vi "Configure Digital Channel.vi"(0 "ADALM2000 In":u32 caption="Instrument Handle Out", 1 "channel":u64 max=15, 2 "Trigger enable":bool, 3 "Output":bool, 4 "Digital Condition":T2, 5 "Cyclic":bool, 7 "Digital Mode":T1, 9 "Digital Delay":i64) -> (14 "ADALM2000 Out":u32 caption="Instrument Handle Out")   [LabVIEW 2015]
uses:
  Controls/DigitalTriggerCondition.ctl
  Controls/DigitalTriggerMode.ctl
  libm2k_lv.dll
panel:
  # "TRIGGER SETTINGS FOR DIO CHANNEL"
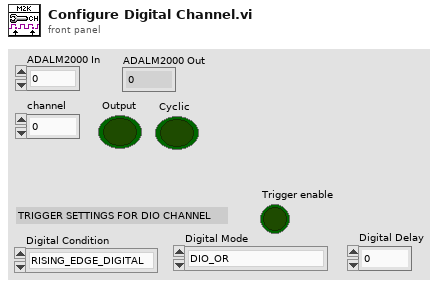
[diagram p1: front panel]
types:
  T1 = typedef "DigitalTriggerMode.ctl" = enum16{"DIO_OR", "DIO_AND"}
  T2 = typedef "DigitalTriggerCondition.ctl" = enum16{"RISING_EDGE_DIGITAL", "FALLING_EDGE_DIGITAL", "LOW_LEVEL_DIGITAL", "HIGH_LEVEL_DIGITAL", "ANY_EDGE_DIGITAL", "NO_TRIGGER_DIGITAL"}
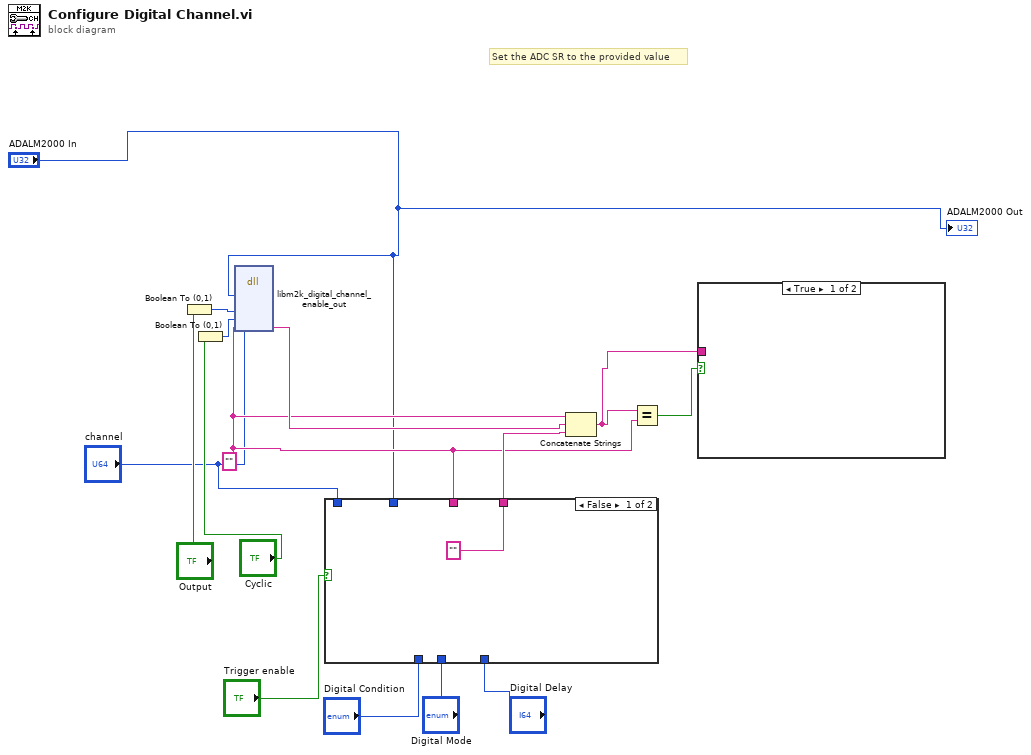
[diagram p0: block diagram]
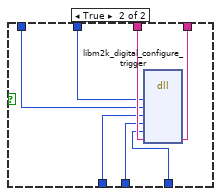
[diagram p2: hidden frame]
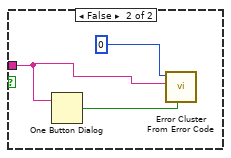
[diagram p3: hidden frame]
diagram:
  w6 = ""
  # "Set the ADC SR to the provided value"
  n1 = Boolean To (0,1)(Boolean="Output") -> (0, 1=w14:i16)
  n2 = Boolean To (0,1)(Boolean="Cyclic") -> (0, 1=w10:i16)
  n3 = dll-call lib="libm2k_lv.*" fn="libm2k_digital_channel_enable_out"("instance"="ADALM2000 In", "channel"="channel", "output"=w14, "cyclic"=w10, "err"=w6) -> ("err"=w11:string)  [unwired: 8 in, 2 out]
  n4 = case shown="False" "Trigger enable" {
    tunnel: ["" w23] -> w7
    tunnel: w6 -> [_ w22]
    tunnel: "ADALM2000 In" -> [_ w21]
    tunnel: "channel" -> [_ w20]
    tunnel: "Digital Condition" -> [_ w19]
    tunnel: "Digital Mode" -> [_ w18]
    tunnel: "Digital Delay" -> [_ w17]
    frame False {
    }
    frame True {
      n5 = dll-call lib="libm2k_lv.*" fn="libm2k_digital_configure_trigger"("instance"=w21, "chnIdx"=w20, "digital_condition"=w19, "digital_mode"=w18, "digital_delay"=w17, "err"=w22) -> ("err"=w23:string)  [unwired: 9 in, 2 out]
    }
  }
  n6 = Concatenate Strings(w6, w11, w7) -> (w12:string)
  n7 = Equal?(x=w12, y=w6) -> (x = y?=w13:bool)
  n8 = case shown="True" w13 {
    tunnel: w12 -> [_ w24]
    frame True {
    }
    frame False {
      n9 = One Button Dialog(message=w24) -> (true=w26:bool)  [unwired: 1 in]
      n10 = call <vilib>:"Error Cluster From Error Code.vi"("show call chain? (False)"=w26, "error message (\"\")"=w24, "error code (0)"=0) -> ()  [unwired: 6 in, 1 out]
    }
  }
  "ADALM2000 Out" <- "ADALM2000 In"
